vi "Gwinstek_chan_1_2.vi"() -> ()   [LabVIEW 2018]
uses:
  Downloads/LVdriver_AFG-2225_V1_E/AFG-2225/AFG-2225.lvlib
panel:
  in  "LOAD Command chan 2":string=";OUTP1:LOAD INF;"
  in  "LOAD Command chan 1":string=";OUTP1:LOAD INF;"
  in  "DC Offset chan 2":dbl format="%.2g"
  in  "Frequency chan2":dbl=1000.0 format="%_7g"
  in  "Vpp chan 2":dbl=3.0 format="%.3g"
  in  "Waveform Function chan2":u16(ring) items=["Sine", "Square", "Pulse", "Ramp", "Noise"]
  in  "Serial Configuration":T1={"Baud Rate"=9600, "Parity"=0, "Data Bits"=8} {"Data Bits" items=["7"=7, "8"=8]; "Parity" items=["None", "Odd", "Even", "Mark", "Space"]; "Baud Rate" items=["300"=300, "600"=600, "1200"=1200, "2400"=2400, "4800"=4800, "9600"=9600, "19200"=19200]}
  in  "DC Offset chan1":dbl
  in  "Frequency chan1":dbl=1000.0
  in  "Vpp chan 1":dbl=0.1
  in  "Waveform chan1":u16(ring) items=["Sine", "Square", "Triangle"]
  in  "VISA resource name":refnum<visa-resource-name>
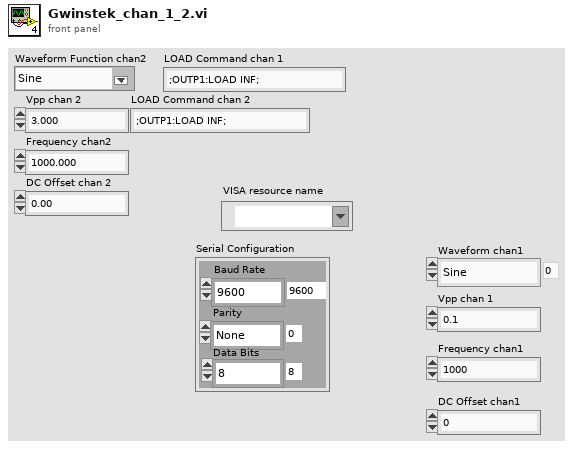
[diagram p1: front panel]
types:
  T1 = cluster{"Baud Rate":u32, "Parity":u16, "Data Bits":u16}
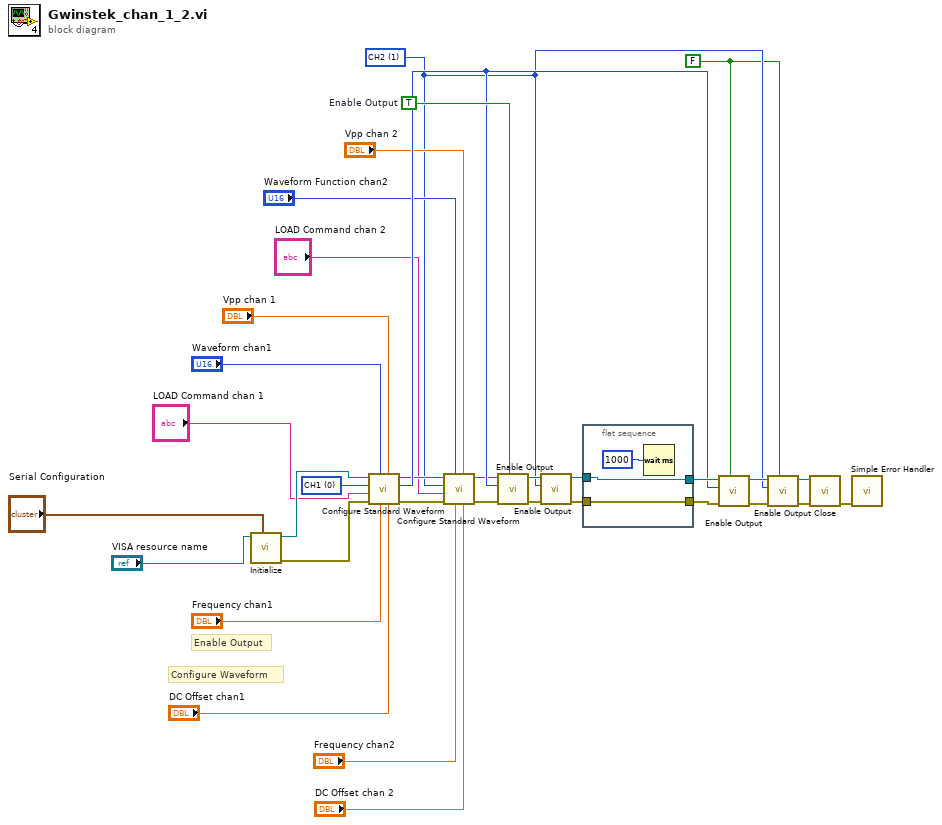
[diagram p0: block diagram]
diagram:
  w6 = u16 1 items=["CH1", "CH2"] ("Channel (0: CH1)")
  w23 = u16 0 items=["CH1", "CH2"] ("Channel (0: CH1)")
  w5 = FALSE ("Enable Output (T: Enable)")
  w30 = TRUE  # Enable Output
  # "Enable Output"
  # "Configure Waveform"
  n1 = call "Initialize.vi"("Serial Configuration"="Serial Configuration", "VISA resource name"="VISA resource name") -> ("error out"=w32:errorcluster, "VISA resource name out"=w33:refnum<visa-resource-name>)  [unwired: 3 in, 5 out]
  n2 = call "Configure Standard Waveform.vi"("DC Offset (0.00 V)"="DC Offset chan1", "Amplitude (3.000 Vpp)"="Vpp chan 1", "Frequency (1000.000 Hz)"="Frequency chan1", "Waveform Function (0: Sine)"="Waveform chan1", "error in (no error)"=w32, "Offset Command"="LOAD Command chan 1", "Channel (0: CH1)"=w23, "VISA resource name"=w33) -> ("error out"=w19:errorcluster, "Channel out"=w24:u16, "VISA resource name out"=w22:refnum<visa-resource-name>)  [unwired: 1 out]
  n3 = call "Configure Standard Waveform.vi"("DC Offset (0.00 V)"="DC Offset chan 2", "Amplitude (3.000 Vpp)"="Vpp chan 2", "Frequency (1000.000 Hz)"="Frequency chan2", "Waveform Function (0: Sine)"="Waveform Function chan2", "error in (no error)"=w19, "Offset Command"="LOAD Command chan 2", "Channel (0: CH1)"=w6, "VISA resource name"=w22) -> ("error out"=w20:errorcluster, "VISA resource name out"=w21:refnum<visa-resource-name>)  [unwired: 2 out]
  n4 = call "Enable Output.vi"("Enable Output (T: Enable)"=w30, "error in (no error)"=w20, "Channel (0: CH1)"=w24, "VISA resource name"=w21) -> ("error out"=w13:errorcluster, "VISA resource name out"=w14:refnum<visa-resource-name>)  [unwired: 6 out]
  n5 = call "Enable Output.vi"("error in (no error)"=w13, "Channel (0: CH1)"=w6, "VISA resource name"=w14) -> ("error out"=w11:errorcluster, "VISA resource name out"=w12:refnum<visa-resource-name>)  [unwired: 1 in, 6 out]
  n6 = flat-sequence {
    tunnel: w12 -> [w36]
    tunnel: w11 -> [w35]
    tunnel: [w36] -> w26
    tunnel: [w35] -> w25
    frame #0 {
      n7 = Wait (ms)(milliseconds to wait=u32 1000) -> ()  [unwired: 1 out]
    }
  }
  n8 = call "Enable Output.vi"("Enable Output (T: Enable)"=w5, "error in (no error)"=w25, "Channel (0: CH1)"=w24, "VISA resource name"=w26) -> ("error out"=w8:errorcluster, "VISA resource name out"=w10:refnum<visa-resource-name>)  [unwired: 6 out]
  n9 = call "Enable Output.vi"("Enable Output (T: Enable)"=w5, "error in (no error)"=w8, "Channel (0: CH1)"=w6, "VISA resource name"=w10) -> ("error out"=w7:errorcluster, "VISA resource name out"=w9:refnum<visa-resource-name>)  [unwired: 6 out]
  n10 = call "Close.vi"("error in (no error)"=w7, "VISA resource name"=w9) -> ("error out"=w31:errorcluster)  [unwired: 9 out]
  n11 = call <vilib>:"Simple Error Handler.vi"("error in (no error)"=w31) -> ()  [unwired: 1 in, 8 out]
